vi "Set Configuration VI XML.vi"(9 "Configuration VI Path":path, 10 "Custom Device Name (No Extension)":string, 11 "Relative Target Location":path) -> (3 "XML String":string)   [LabVIEW 2020, in "Custom Device Template Tool.lvlib"]
uses:
  <vilib>/NI VeriStand/Custom Device Tools/Custom Device Template Tool/Custom Device Template Tool.lvlib
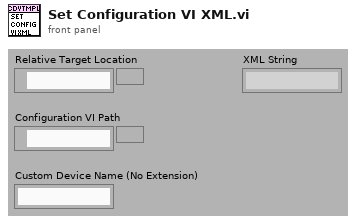
[diagram p1: front panel]
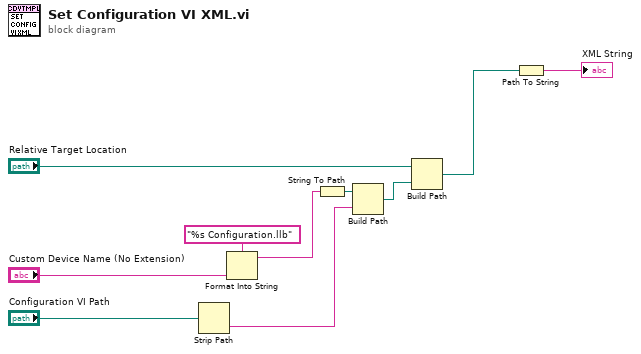
[diagram p0: block diagram]
diagram:
  n1 = Strip Path(path="Configuration VI Path") -> (name=w1:string)  [unwired: 1 out]
  n2 = Format Into String(format string="%s Configuration.llb", "Custom Device Name (No Extension)") -> (resulting string=w5:string)  [unwired: 2 in, 1 out]
  n3 = String To Path(string=w5) -> (path=w6:path)
  n4 = Build Path(base path=w6, name or relative path=w1) -> (appended path=w7:path)
  n5 = Build Path(base path="Relative Target Location", name or relative path=w7) -> (appended path=w8:path)
  n6 = Path To String(path=w8) -> (string=→"XML String":string)
